vi "Práctica7.2_DAQ 6210.vi"() -> ()   [LabVIEW 2018]
panel:
  out "Entrada analógica":dbl(knob) scale=0.0..5.0
  out "Entradas digitales":bool[](array[boolean])
  in  "Alto":bool
  in  "Salidas digitales":bool[](array[boolean])
  # "Anahí Montserrat Vázquez Padilla\nMiércoles 13 de marzo del 2024 \nPráctica 8. DAQ 2610"
  # "Valeria Padilla Sandoval\nIMEC 218480301\n\nPráctica X. \nComunicación DAQ"
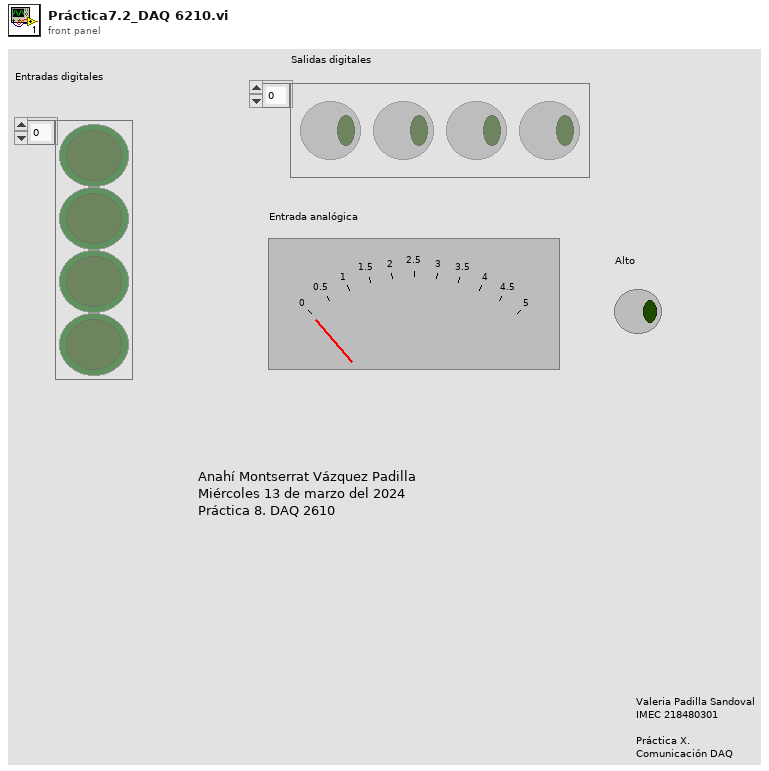
[diagram p1: front panel]
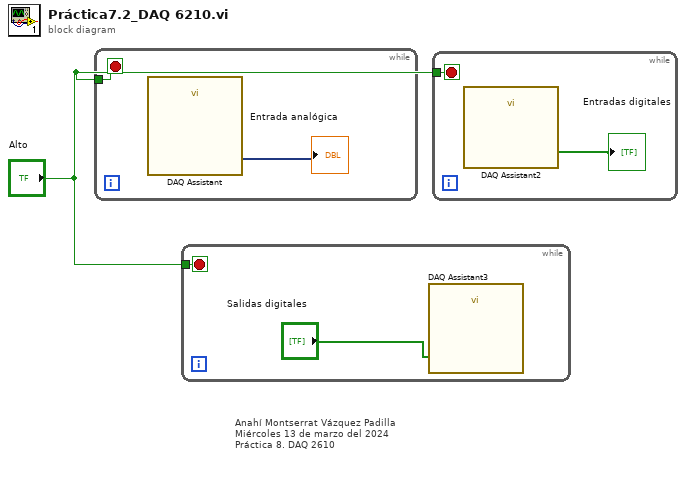
[diagram p0: block diagram]
diagram:
  # "Anahí Montserrat Vázquez Padilla\nMiércoles 13 de marzo del 2024 \nPráctica 8. DAQ 2610"
  n1 = while {
    tunnel: "Alto" -> [w3]
    stop <- w3 stop-if-true
    n2 = call "DAQ Assistant"() -> ("data"=→"Entrada analógica":dynamicdata)  [unwired: 17 in, 2 out]
  }
  n3 = while {
    tunnel: "Alto" -> [w5]
    stop <- w5 stop-if-true
    n4 = call "DAQ Assistant3"("data"="Salidas digitales") -> ()  [unwired: 17 in, 2 out]
  }
  n5 = while {
    tunnel: "Alto" -> [w7]
    stop <- w7 stop-if-true
    n6 = call "DAQ Assistant2"() -> ("data"=→"Entradas digitales":bool[])  [unwired: 17 in, 2 out]
  }
